vi "CSM - System States.vi"() -> (3 "items to filter":string[](array[string]))   [LabVIEW 2017, in "CSM Shared.lvlib"]
uses:
  CSM Shared.lvlib
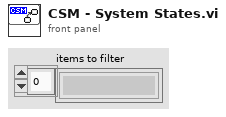
[diagram p1: front panel]
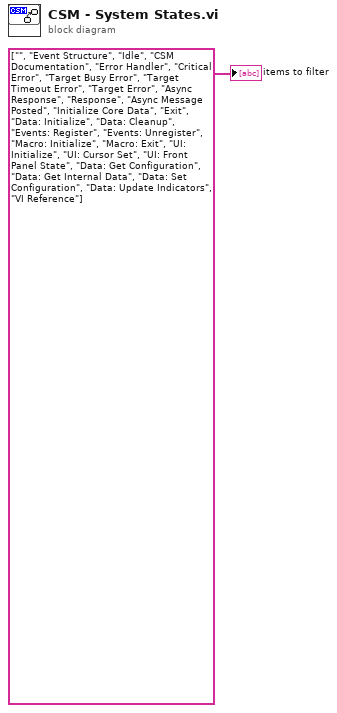
[diagram p0: block diagram]
diagram:
  "items to filter" <- string[] ["", "Event Structure", "Idle", "CSM Documentation", "Error Handler", "Critical Error", "Target Busy Error", "Target Timeout Error", "Target Error", "Async Response", "Response", "Async Message Posted", "Initialize Core Data", "Exit", "Data: Initialize", "Data: Cleanup", "Events: Register", "Events: Unregister", "Macro: Initialize", "Macro: Exit", "UI: Initialize", "UI: Cursor Set", "UI: Front Panel State", "Data: Get Configuration", "Data: Get Internal Data", "Data: Set Configuration", "Data: Update Indicators", "VI Reference"] ("items to filter")
